vi "Configure Dialog.vi"(8 "Error In":errorcluster, 11 "Auto Mute Msg in":refnum<class "Auto Mute Msg.lvclass">) -> (0 "Error Out":errorcluster, 2 "OK?":bool, 3 "Auto Mute Msg out":refnum<class "Auto Mute Msg.lvclass">)   [LabVIEW 2014, in "KIT-QVA.lvlib" / "Auto Mute Msg.lvclass"]
doc: "This overrides of this dynamic dispatch VI open the frontpanel to set derived message attributes."
uses:
  Auto Mute Msg.lvclass
  Auto Mute Msg.lvclass/Auto Mute Msg.ctl
panel:
  in  "Auto Mute":bool
  in  "OK":bool
  in  "Cancel":bool
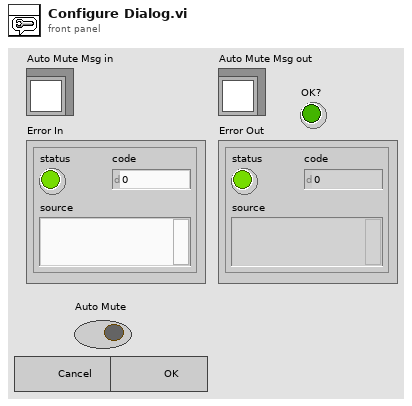
[diagram p1: front panel]
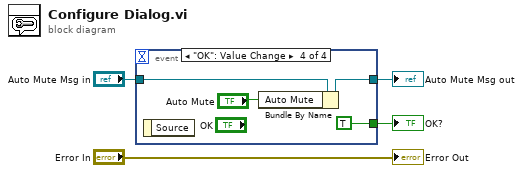
[diagram p0: block diagram]
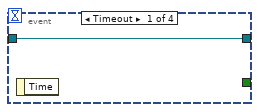
[diagram p2: hidden frame]
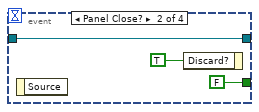
[diagram p3: hidden frame]
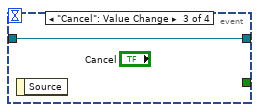
[diagram p4: hidden frame]
diagram:
  n1 = event shown="[3] \"OK\": Value Change" {
    selector: _ -> [_ _ _ _]
    dyn-events: _ -> [_ _ _ _]
    timeout: _ -> [_ _ _ _]
    tunnel: [w5 w6 w9 w12] -> w2
    tunnel: "Auto Mute Msg in" -> [w5 w6 w9 w13]
    tunnel: [_ FALSE _ TRUE] -> w1
    event Timeout {
      n2 = event-data() -> ()  [unwired: 1 in, 1 out]
    }
    event Panel Close? {
      n3 = event-data() -> ()  [unwired: 1 in, 1 out]
      n4 = event-data("Discard?"=TRUE) -> ()  [unwired: 1 in, 1 out]
    }
    event "Cancel": Value Change {
      n5 = event-data() -> ()  [unwired: 1 in, 1 out]
    }
    event "OK": Value Change {
      n6 = event-data() -> ()  [unwired: 1 in, 1 out]
      n7 = Bundle By Name(cluster=w13, "Auto Mute"="Auto Mute") -> (w12:refnum<class "Auto Mute Msg.lvclass">)
    }
  }
  "Auto Mute Msg out" <- w2
  "OK?" <- w1
  "Error Out" <- "Error In"
